vi "TankDrive.vi"(9 "Right Stick":dbl, 10 "Left Stick":dbl, 11 "Cluster of Drive Def Refs":T5) -> (1 "Right Motor Value":dbl, 2 "Left Motor Value":dbl, 3 "Cluster of Drive Def Refs Out":T5)   [LabVIEW 2016]
uses:
  <vilib>/Rock Robotics/WPI/MotorControl/WPI_MotorControlDeviceRef.ctl
  <vilib>/Rock Robotics/WPI/MotorControl/WPI_MotorControlType.ctl
  <vilib>/Rock Robotics/SystemInterfaces/DIO/FPGA_DIOPWMChannel.ctl
  <vilib>/Rock Robotics/WPI/PWM/WPI_PWMDeadband.ctl
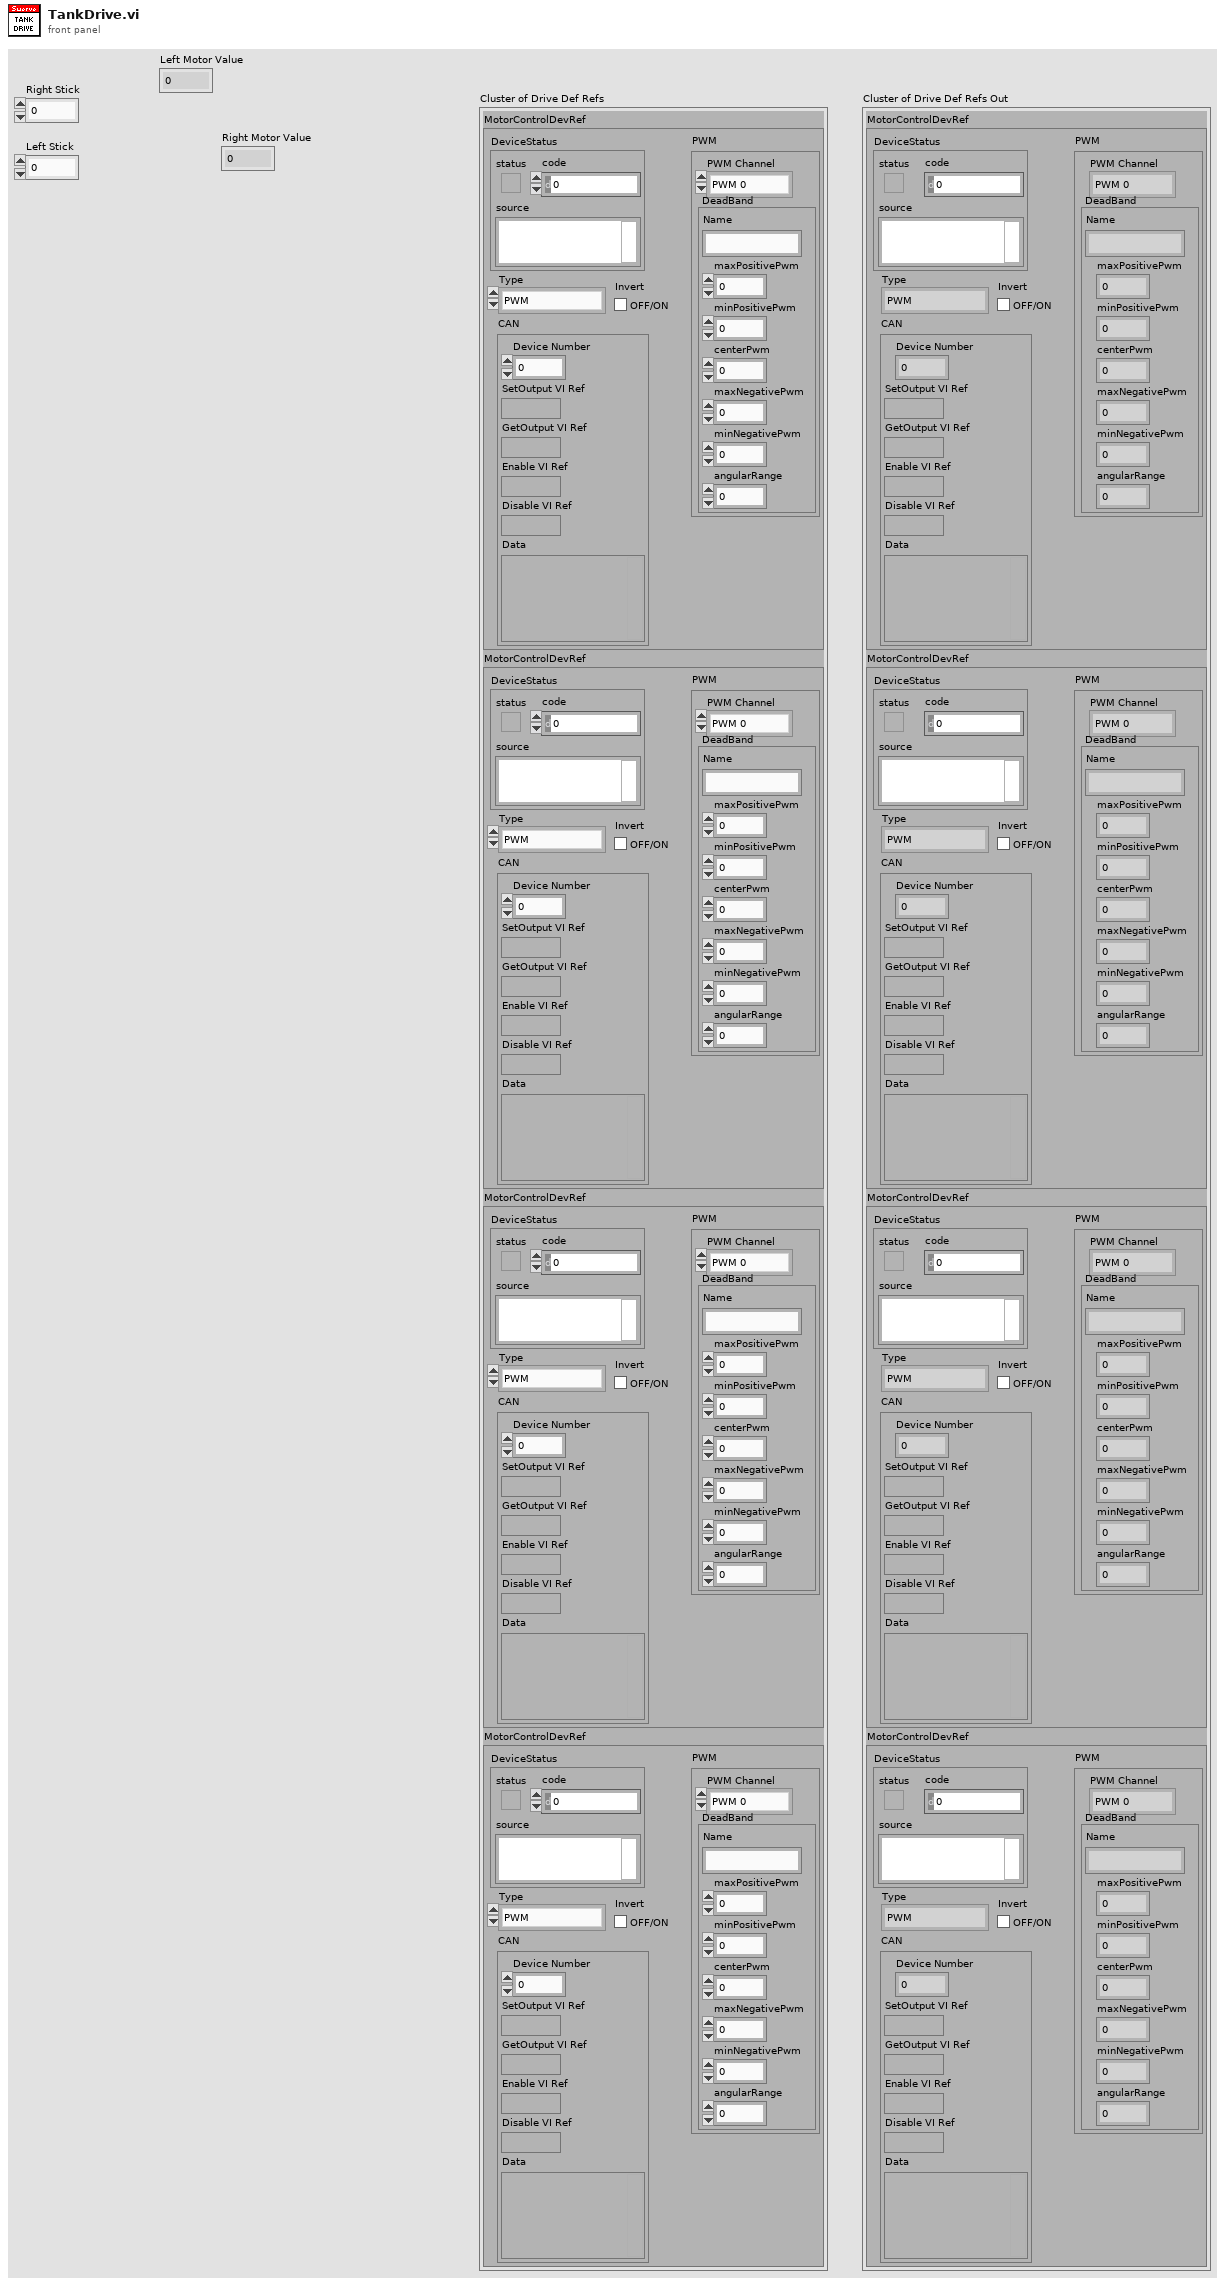
[diagram p1: front panel]
types:
  T1 = typedef "WPI_MotorControlDeviceRef.ctl" = cluster{"DeviceStatus":errorcluster, "Type":T2, "PWM":cluster{"PWM Channel":T3, "DeadBand":T4}, "CAN":cluster{"Device Number":u8, "SetOutput VI Ref":variant, "GetOutput VI Ref":variant, "Enable VI Ref":variant, "Disable VI Ref":variant, "Data":variant}, "Invert":bool}
  T2 = typedef "WPI_MotorControlType.ctl" = enum16{"PWM", "CAN"}
  T3 = typedef "FPGA_DIOPWMChannel.ctl" = enum8{"PWM 0", "PWM 1", "PWM 2", "PWM 3", "PWM 4", "PWM 5", "PWM 6", "PWM 7", "PWM 8", "PWM 9", "PWM MXP 0", "PWM MXP 1", "PWM MXP 2", "PWM MXP 3", "PWM MXP 4", "PWM MXP 5", "PWM MXP 6", "PWM MXP 7", "PWM MXP 8", "PWM MXP 9", "Invalid"}
  T4 = typedef "WPI_PWMDeadband.ctl" = cluster{"Name":string, "maxPositivePwm":i32, "minPositivePwm":i32, "centerPwm":i32, "maxNegativePwm":i32, "minNegativePwm":i32, "angularRange":u16}
  T5 = cluster{"MotorControlDevRef":T1, "MotorControlDevRef":T1, "MotorControlDevRef":T1, "MotorControlDevRef":T1}
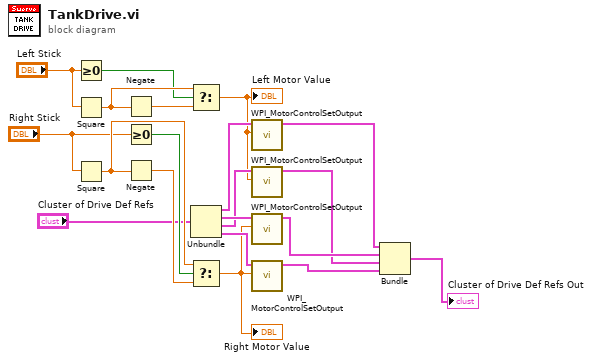
[diagram p0: block diagram]
diagram:
  n1 = Greater Or Equal To 0?(x="Left Stick") -> (x >= 0?=w14:bool)
  n2 = Square(x="Left Stick") -> (x^2=w15:dbl)
  n3 = Square(x="Right Stick") -> (x^2=w20:dbl)
  n4 = Negate(x=w15) -> (-x=w16:dbl)
  n5 = Greater Or Equal To 0?(x="Right Stick") -> (x >= 0?=w19:bool)
  n6 = Negate(x=w20) -> (-x=w18:dbl)
  n7 = Select(t=w15, s=w14, f=w16) -> (s? t:f=w7:dbl)
  "Left Motor Value" <- w7
  n8 = Unbundle("Cluster of Drive Def Refs") -> ("MotorControlDevRef"=w11:T1, "MotorControlDevRef"=w10:T1, "MotorControlDevRef"=w9:T1, "MotorControlDevRef"=w8:T1)
  n9 = Select(t=w20, s=w19, f=w18) -> (s? t:f=w6:dbl)
  "Right Motor Value" <- w6
  n10 = call <vilib>:"WPI_MotorControlSetOutput.vi"("Output"=w7, "MotorControlDevRef"=w11) -> ("MotorControlDevRef"=w5:T1)  [unwired: 7 in, 2 out]
  n11 = call <vilib>:"WPI_MotorControlSetOutput.vi"("Output"=w7, "MotorControlDevRef"=w9) -> ("MotorControlDevRef"=w3:T1)  [unwired: 7 in, 2 out]
  n12 = call <vilib>:"WPI_MotorControlSetOutput.vi"("Output"=w6, "MotorControlDevRef"=w10) -> ("MotorControlDevRef"=w4:T1)  [unwired: 7 in, 2 out]
  n13 = call <vilib>:"WPI_MotorControlSetOutput.vi"("Output"=w6, "MotorControlDevRef"=w8) -> ("MotorControlDevRef"=w2:T1)  [unwired: 7 in, 2 out]
  n14 = Bundle("MotorControlDevRef"=w5, "MotorControlDevRef"=w4, "MotorControlDevRef"=w3, "MotorControlDevRef"=w2) -> (→"Cluster of Drive Def Refs Out":T5)  [unwired: 1 in]
